vi "dilutionCalc.vi"(4 "Calculated":u16, 6 "MFC3":dbl, 7 "MFC2":dbl, 8 "MFC1":dbl, 9 "flow":dbl) -> (0 "MFC3 out":dbl, 1 "MFC2 out":dbl, 2 "MFC1 out":dbl, 3 "flow out":dbl)   [LabVIEW 2011]
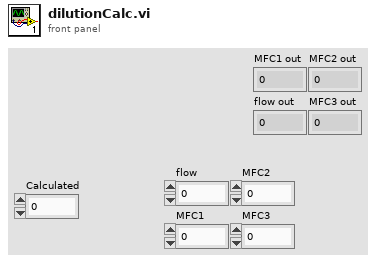
[diagram p1: front panel]
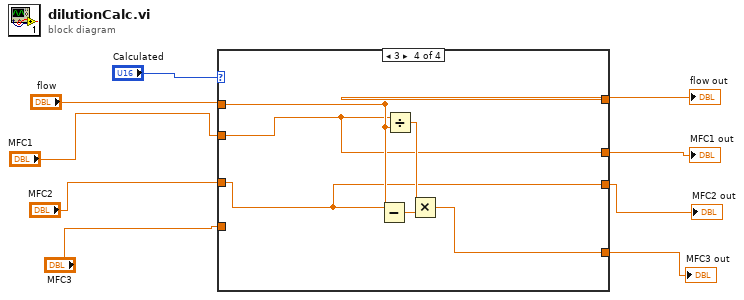
[diagram p0: block diagram]
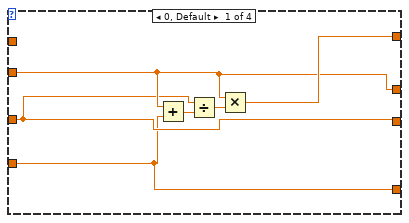
[diagram p2: hidden frame]
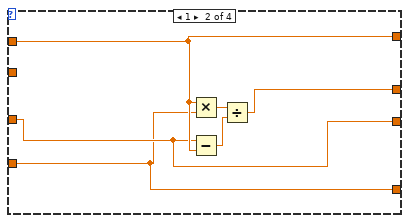
[diagram p3: hidden frame]
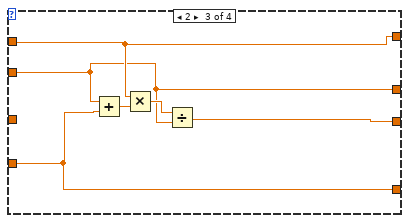
[diagram p4: hidden frame]
diagram:
  n1 = case shown="3" "Calculated" {
    tunnel: "flow" -> [_ w18 w24 w30]
    tunnel: [w13 w18 w24 w30] -> w8
    tunnel: "MFC1" -> [w12 _ w23 w29]
    tunnel: "MFC3" -> [w10 w16 w22 _]
    tunnel: "MFC2" -> [w11 w17 _ w28]
    tunnel: [w12 w19 w23 w29] -> w3
    tunnel: [w11 w17 w25 w28] -> w2
    tunnel: [w10 w16 w22 w31] -> w1
    frame 0, Default {
      n2 = Add(x=w12, y=w10) -> (x+y=w14:dbl)
      n3 = Divide(x=w11, y=w14) -> (x/y=w15:dbl)
      n4 = Multiply(x=w12, y=w15) -> (x*y=w13:dbl)
    }
    frame 1 {
      n5 = Multiply(x=w18, y=w16) -> (x*y=w21:dbl)
      n6 = Subtract(x=w17, y=w18) -> (x-y=w20:dbl)
      n7 = Divide(x=w21, y=w20) -> (x/y=w19:dbl)
    }
    frame 2 {
      n8 = Add(x=w23, y=w22) -> (x+y=w27:dbl)
      n9 = Multiply(x=w24, y=w27) -> (x*y=w26:dbl)
      n10 = Divide(x=w26, y=w23) -> (x/y=w25:dbl)
    }
    frame 3 {
      n11 = Subtract(x=w28, y=w30) -> (x-y=w32:dbl)
      n12 = Divide(x=w29, y=w30) -> (x/y=w33:dbl)
      n13 = Multiply(x=w33, y=w32) -> (x*y=w31:dbl)
    }
  }
  "flow out" <- w8
  "MFC1 out" <- w3
  "MFC2 out" <- w2
  "MFC3 out" <- w1
